vi "_DServerRequestDataToStateScalar.vi"(0 "client request":T2={"Request Id"=0, "Source Id"=0, "Request Type"=enum."UNKNOWN_REQUEST", "Device Class Name"="unspecified_class_name", "Device Name"="unspecified/device/name", "Cmd or Attr Name"="unspecified_cmd_or_attr_name", "Client Request Data"={"write attribute value"={"dimx"=0, "dimy"=0, "data"=[], "data_type"=enum."UNKNOWN_DATA_TYPE"}, "exec. command argin"={"num data"=[], "str data"=[]}}}) -> (1 "attribute value":T1=enum."UNKNOWN", 2 "client request":T2={"Request Id"=0, "Source Id"=0, "Request Type"=enum."UNKNOWN_REQUEST", "Device Class Name"="unspecified_class_name", "Device Name"="unspecified/device/name", "Cmd or Attr Name"="unspecified_cmd_or_attr_name", "Client Request Data"={"write attribute value"={"dimx"=0, "dimy"=0, "data"=[], "data_type"=enum."UNKNOWN_DATA_TYPE"}, "exec. command argin"={"num data"=[], "str data"=[]}}})   [LabVIEW 2014, in "tango.lvlib"]
uses:
  tango.lvlib
  Client Request Handling/Typedefs/_DServerClientRequest.ctl
  Client Request Handling/Typedefs/_DServerClientRequestType.ctl
  Client Request Handling/Typedefs/_DServerClientRequestData.ctl
  Typedefs/_GenericDataBuffer.ctl
  Common VIs/Typedefs/_AttributeDataType_t.ctl
  Common VIs/Typedefs/_TangoState_t.ctl
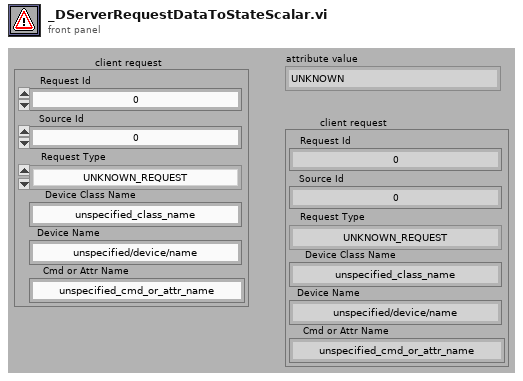
[diagram p1: front panel]
types:
  T1 = typedef "tango.lvlib/_TangoState_t.ctl" = enum32{"ON", "OFF", "CLOSE", "OPEN", "INSERT", "EXTRACT", "MOVING", "STANDBY", "FAULT", "INIT", "RUNNING", "ALARM", "DISABLE", "UNKNOWN"}
  T2 = typedef "tango.lvlib/_DServerClientRequest.ctl" = cluster{"Request Id":u32, "Source Id":u32, "Request Type":T3, "Device Class Name":string, "Device Name":string, "Cmd or Attr Name":string, "Client Request Data":T4}
  T3 = typedef "tango.lvlib/_DServerClientRequestType.ctl" = enum16{"EXEC_CMD", "READ_ATTR", "WRITE_ATTR", "UNKNOWN_REQUEST"}
  T4 = typedef "tango.lvlib/_DServerClientRequestData.ctl" = cluster{"write attribute value":T5, "exec. command argin":cluster{"num data":u8[], "str data":string[]}}
  T5 = typedef "tango.lvlib/_GenericDataBuffer.ctl" = cluster{"dimx":u32, "dimy":u32, "data":u8[], "data_type":T6}
  T6 = typedef "tango.lvlib/_AttributeDataType_t.ctl" = enum16{"STATE_SCA", "STATE_SPE", "STATE_IMG", "STRING_SCA", "STRING_SPE", "STRING_IMG", "BOOL_SCA", "BOOL_SPE", "BOOL_IMG", "UCHAR_SCA", "UCHAR_SPE", "UCHAR_IMG", "SHORT_SCA", "SHORT_SPE", "SHORT_IMG", "USHORT_SCA", "USHORT_SPE", "USHORT_IMG", "LONG_SCA", "LONG_SPE", "LONG_IMG", "ULONG_SCA", "ULONG_SPE", "ULONG_IMG", "LONG64_SCA", "LONG64_SPE", "LONG64_IMG", "ULONG64_SCA", "ULONG64_SPE", "ULONG64_IMG", "FLOAT_SCA", "FLOAT_SPE", "FLOAT_IMG", "DOUBLE_SCA", "DOUBLE_SPE", "DOUBLE_IMG", "UNKNOWN_DATA_TYPE"}
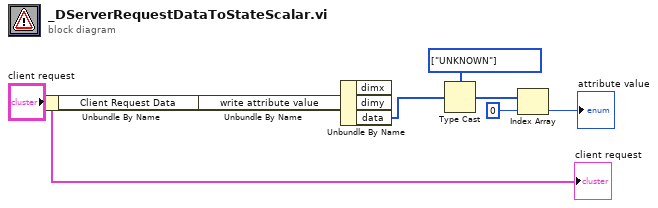
[diagram p0: block diagram]
diagram:
  w8 = T1[] [enum."UNKNOWN"] items=["ON", "OFF", "CLOSE", "OPEN", "INSERT", "EXTRACT", "MOVING", "STANDBY", "FAULT", "INIT", "RUNNING", "ALARM", "DISABLE", "UNKNOWN"]
  n1 = Unbundle By Name("client request") -> ("Client Request Data"=w5:T4)
  n2 = Unbundle By Name(w5) -> ("write attribute value"=w4:T5)
  n3 = Unbundle By Name(w4) -> ("data"=w3:u8[])  [unwired: 2 out]
  n4 = Type Cast(type=w8, x=w3) -> (*(type *) &x=w6:T1[])
  n5 = Index Array(array=w6, index=0 ("indice")) -> (element=→"attribute value":T1)
  "client request" <- "client request"
